vi "New Error.vi"(7 "vi name":string, 11 "error":T1) -> (1 "initial offset":i32, 3 "error":errorcluster)   [LabVIEW 2017, in "PXImc.lvlib" / "PXImc Transceiver.lvclass"]
uses:
  PXImc Transceiver.lvclass
  Errors.ctl
  <vilib>/NI/Memory Manager/VIs/New Error Cluster (512B).vi
  <vilib>/NI/Memory Manager/Static Errors.lvlib
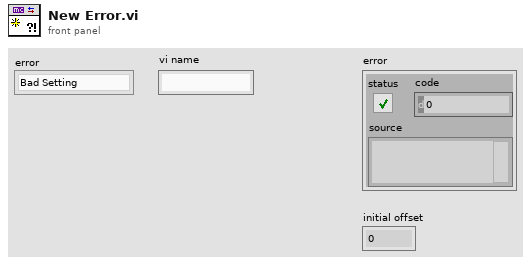
[diagram p1: front panel]
types:
  T1 = typedef "PXImc.lvlib/PXImc Transceiver.lvclass/Errors.ctl" = enum8{"Bad Setting", "Duplicate Stream ID"}
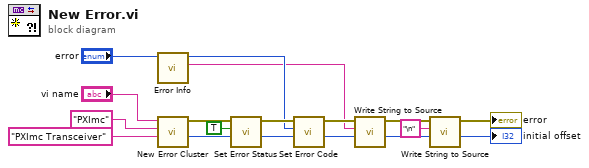
[diagram p0: block diagram]
diagram:
  n1 = call "Error Info.vi"("error"="error") -> ("description"=w6:string, "code"=w9:i32)  [unwired: 9 in]
  n2 = call-poly <vilib>:"New Error Cluster.vi"("class name (\"\")"="PXImc Transceiver" ("class name (\"\")"), "library name (\"\")"="PXImc" ("library name (\"\")"), "vi name (\"\")"="vi name") -> ("initial offset"=w13:i32, "error out"=w14:errorcluster)  [unwired: 7 in]
  n3 = call <vilib>:"Set Error Status.vi"("offset"=w13, "status (T)"=TRUE, "error in"=w14) -> ("offset"=w11:i32, "error out"=w10:errorcluster)  [unwired: 7 in]
  n4 = call <vilib>:"Set Error Code.vi"("offset"=w11, "code"=w9, "error in"=w10) -> ("offset"=w7:i32, "error out"=w8:errorcluster)  [unwired: 7 in]
  n5 = call <vilib>:"Write String to Source.vi"("offset"=w7, "string"=w6, "error in"=w8) -> ("new offset"=w4:i32, "error out"=w5:errorcluster)  [unwired: 7 in]
  n6 = call <vilib>:"Write String to Source.vi"("offset"=w4, "string"="\n", "error in"=w5) -> ("new offset"=→"initial offset":i32, "error out"=→"error":errorcluster)  [unwired: 7 in]
